vi "1D String Array to String.vi"(6 "Delimiter (,)":string=",", 8 "error in (no error)":errorcluster, 11 "1D Array[]":string[](array[string])) -> (0 "error out":errorcluster, 3 "String":string)   [LabVIEW 2016, in "SLL String.lvlib"]
uses:
  SLL String.lvlib
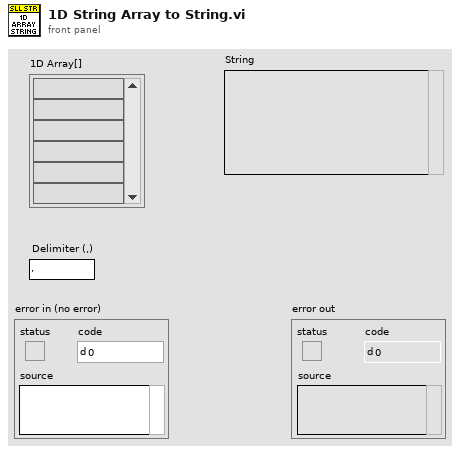
[diagram p1: front panel]
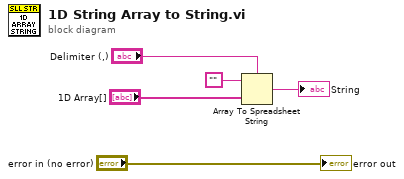
[diagram p0: block diagram]
diagram:
  n1 = Array To Spreadsheet String(delimiter (Tab)="Delimiter (,)", array="1D Array[]", 3:"") -> (spreadsheet string=→"String":string)
  "error out" <- "error in (no error)"
